vi "Save JWT to File.vi"(8 "error in (no error)":errorcluster, 9 "Replace? (F)":bool, 10 "JWT":string, 11 "JWT Path In":path) -> (0 "error out":errorcluster, 3 "JWT Path":path)   [LabVIEW 2020, in "JWT.lvlib"]
uses:
  JWT.lvlib
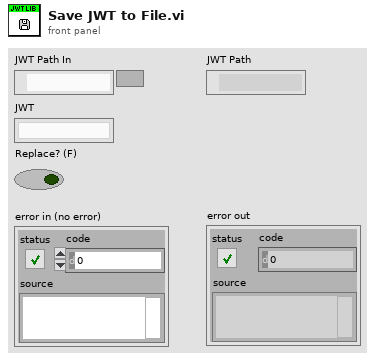
[diagram p1: front panel]
types:
  T1 = enum16{"open", "replace", "create", "open or create", "replace or create", "replace or create with confirmation"}
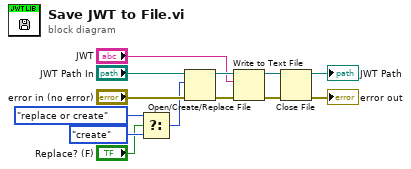
[diagram p0: block diagram]
diagram:
  n1 = Select(t=T1."replace or create" ("operation (0:open)"), s="Replace? (F)", f=T1."create" ("operation (0:open)")) -> (s? t:f=w9:T1)
  n2 = Open/Create/Replace File(file path (use dialog)="JWT Path In", error in="error in (no error)", operation (0:open)=w9) -> (refnum out=w6:refnum<file>, error out=w7:errorcluster)  [unwired: 3 in, 1 out]
  n3 = Write to Text File(file (use dialog)=w6, text="JWT", error in=w7) -> (refnum out=w3:refnum<file>, error out=w4:errorcluster)  [unwired: 1 in, 1 out]
  n4 = Close File(refnum=w3, error in=w4) -> (path=→"JWT Path":path, error out=→"error out":errorcluster)
